vi "ConvertTo(RunTest).vi"(8 "error in":errorcluster, 9 "Message Payload":variant) -> (0 "error out":errorcluster, 1 "RunTest":T1)   [LabVIEW 2019]
doc: "Convert variant to DAQmx waveform type\n\nBolder Software LLC"
uses:
  RunTest.ctl
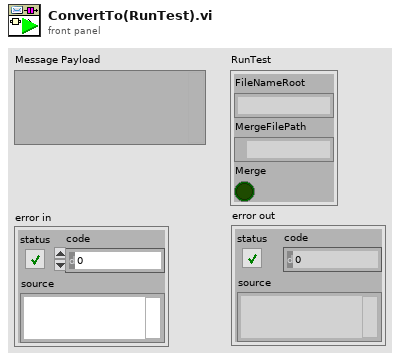
[diagram p1: front panel]
types:
  T1 = typedef "RunTest.ctl" = cluster{"FileNameRoot":string, "MergeFilePath":path, "Merge":bool}
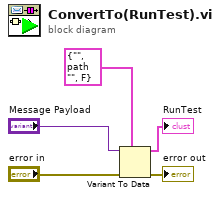
[diagram p0: block diagram]
diagram:
  n1 = Variant To Data(error in="error in", type=T1 {"FileNameRoot"="", "MergeFilePath"=path "", "Merge"=FALSE} ("RunTest"), Variant="Message Payload") -> (data=→"RunTest":T1, error out=→"error out":errorcluster)
